vi "Create Channel.vi"(6 "index":i32, 8 "error in":errorcluster, 10 "settings":T1={"name"="", "default value"=0.0, "thermocouple type"=enum."J", "measurement units"=enum."Degrees Celsius"}, 11 "thermocouple mode in":refnum<class "Thermocouple Mode.lvclass">) -> (0 "error out":errorcluster, 2 "thermocouple channel out":refnum<class "Thermocouple Channel.lvclass">, 3 "thermocouple mode out":refnum<class "Thermocouple Mode.lvclass">)   [LabVIEW 2017, in "Scan Engine Scripting.lvlib" / "Thermocouple Mode.lvclass"]
doc: "Creates an instance of a channel."
uses:
  Thermocouple Mode.lvclass
  Controls/thermocouple channel settings.ctl
  Channel Classes/Thermocouple Channel/Thermocouple Type.ctl
  Channel Classes/Thermocouple Channel/Measurement Units.ctl
  Channel Classes/Thermocouple Channel/Thermocouple Channel.lvclass
  Channel Classes/Thermocouple Channel/Thermocouple Channel Settings.ctl
  Thermocouple Mode.lvclass/Thermocouple Mode.ctl
  Scan Engine Scripting.lvlib
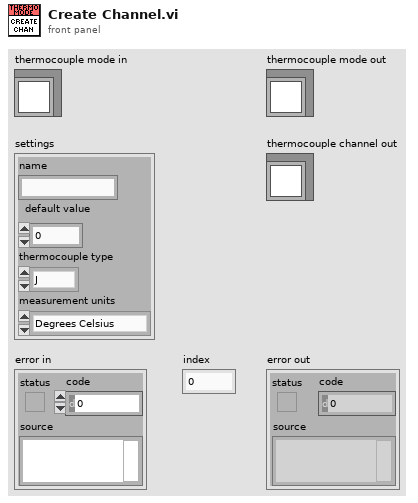
[diagram p1: front panel]
types:
  T1 = typedef "Scan Engine Scripting.lvlib/thermocouple channel settings.ctl" = cluster{"name":string, "default value":dbl, "thermocouple type":T2, "measurement units":T3}
  T2 = typedef "Scan Engine Scripting.lvlib/Thermocouple Channel.lvclass/Thermocouple Type.ctl" = enum16{"J", "K", "T", "E", "R", "S", "N", "B"}
  T3 = typedef "Scan Engine Scripting.lvlib/Thermocouple Channel.lvclass/Measurement Units.ctl" = enum16{"Raw Volts", "Degrees Kelvin", "Degrees Celsius", "Degrees Fahrenheit", "Degrees Rankine"}
  T4 = typedef "Scan Engine Scripting.lvlib/Thermocouple Channel.lvclass/Thermocouple Channel Settings.ctl" = cluster{"thermocouple type":T2, "measurement units":T3}
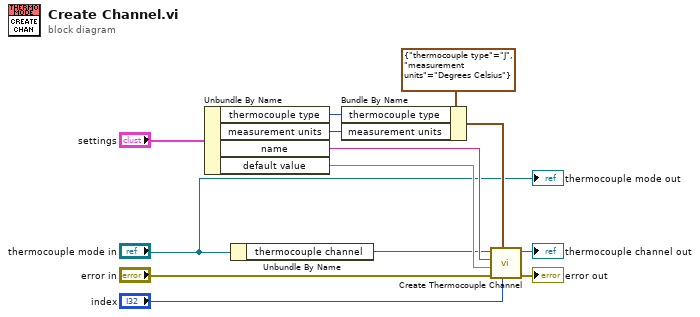
[diagram p0: block diagram]
diagram:
  n1 = Unbundle By Name("settings") -> ("thermocouple type"=w6:T2, "measurement units"=w5:T3, "name"=w10:string, "default value"=w9:dbl)
  n2 = Unbundle By Name("thermocouple mode in") -> ("thermocouple channel"=w3:refnum<class "Thermocouple Channel.lvclass">)
  n3 = Bundle By Name(cluster=T4 {"thermocouple type"=enum."J", "measurement units"=enum."Degrees Celsius"} ("thermocouple channel settings"), "thermocouple type"=w6, "measurement units"=w5) -> (w4:T4)
  n4 = call "Create Thermocouple Channel.vi"("index"="index", "thermocouple channel settings"=w4, "error in"="error in", "default value"=w9, "name"=w10, "thermocouple channel in"=w3) -> ("error out"=→"error out":errorcluster, "thermocouple channel out"=→"thermocouple channel out":refnum<class "Thermocouple Channel.lvclass">)  [unwired: 4 in]
  "thermocouple mode out" <- "thermocouple mode in"
